vi "convertPositionResponse.vi"(8 "error in (no error)":errorcluster, 10 "maxLength":dbl, 11 "pData":u8[](array[numeric])) -> (0 "error out":errorcluster, 1 "cmd":u8, 2 "position":dbl, 3 "rawDataOut":u8[](array[numeric]))   [LabVIEW 2019]
doc: "Scale actuator value to millimeters\n\n(Distance / Stroke )× 1023\n\nFormat: 3-byte packet\nControl, Data Low, Data High\nBuffer[0]=Control\nBuffer[1]=Data Low\nBuffer[2]=Data High\n\n\n\nWritten by: Complete Automated Solutions\nwww.CompleteAutomatedSolutions.com"
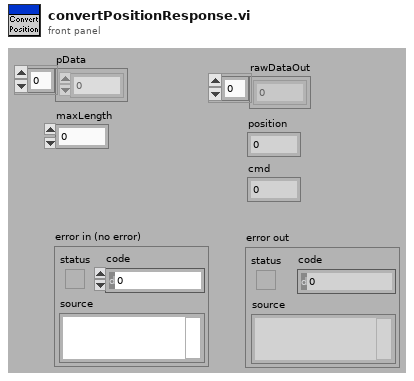
[diagram p1: front panel]
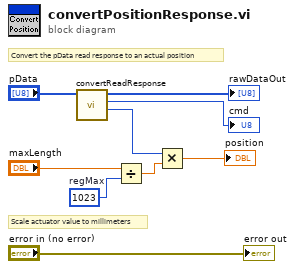
[diagram p0: block diagram]
diagram:
  w8 = u16 1023  # regMax
  # "Scale actuator value to millimeters"
  # "Convert the pData read response to an actual position"
  n1 = call "convertReadResponse.vi"("rawDataIn"="pData") -> ("setValue"=w9:u16, "cmd"=→"cmd":u8, "rawDataOut"=→"rawDataOut":u8[])  [unwired: 1 in, 7 out]
  n2 = Divide(x="maxLength", y=w8) -> (x/y=w6:dbl)
  n3 = Multiply(x=w9, y=w6) -> (x*y=→"position":dbl)
  "error out" <- "error in (no error)"
